vi "FancyPID.vi"(4 "Reset":bool, 6 "Gains":T1={"proportional gain (Kc)"=1.0, "integral time (Ti, min)"=0.01, "derivative time (Td, min)"=0.0} {"derivative time (Td, min)" format="%.3f"; "integral time (Ti, min)" format="%.3f"; "proportional gain (Kc)" format="%.3f"}, 7 "Range":cluster{"output high":dbl, "output low":dbl}={"output high"=0.6, "output low"=-0.6} {"output low" format="%.2f"; "output high" format="%.2f"}, 8 "Disable Range":dbl=0.5, 9 "Integral Range":dbl=25.0, 10 "Process variable":dbl, 11 "Setpoint":dbl) -> (3 "output":dbl format="%.2f")   [LabVIEW 2016]
uses:
  <vilib>/addons/control/pid/pid.llb/PID (DBL).vi
  <vilib>/addons/control/pid/NI_PID_pid.lvlib
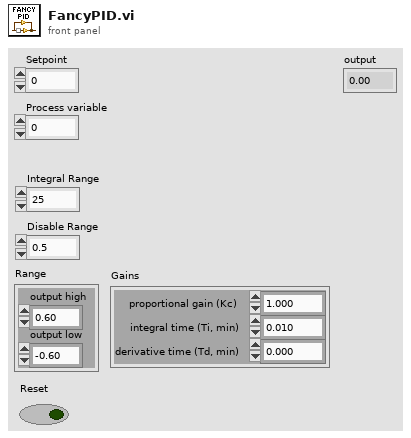
[diagram p1: front panel]
types:
  T1 = cluster{"proportional gain (Kc)":dbl, "integral time (Ti, min)":dbl, "derivative time (Td, min)":dbl}
  T2 = cluster{"proportional gain (Kc)":dbl, "f":dbl, "derivative time (Td, min)":dbl}
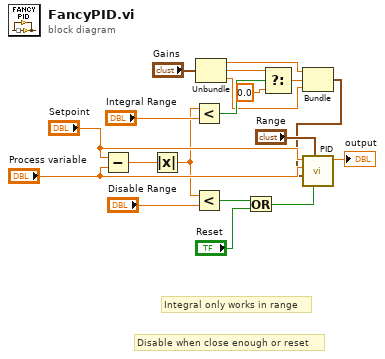
[diagram p0: block diagram]
diagram:
  # "Disable when close enough or reset"
  # "Integral only works in range"
  n1 = Subtract(x="Setpoint", y="Process variable") -> (x-y=w15:dbl)
  n2 = Absolute Value(x=w15) -> (abs(x)=w5:dbl)
  n3 = Less?(x=w5, y="Integral Range") -> (x < y?=w13:bool)
  n4 = Less?(x=w5, y="Disable Range") -> (x < y?=w3:bool)
  n5 = Unbundle("Gains") -> ("proportional gain (Kc)"=w8:dbl, "integral time (Ti, min)"=w11:dbl, "derivative time (Td, min)"=w7:dbl)
  n6 = Or(x=w3, y="Reset") -> (x .or. y?=w2:bool)
  n7 = Select(t=w11, s=w13, f=0.0) -> (s? t:f=w9:dbl)
  n8 = Bundle("proportional gain (Kc)"=w8, "f"=w9, "derivative time (Td, min)"=w7) -> (w1:T2)  [unwired: 1 in]
  n9 = call-poly <vilib>:"PID.vi"("reinitialize? (F)"=w2, "output range"="Range", "PID gains"=w1, "process variable"="Process variable", "setpoint"="Setpoint") -> ("output"=→"output":dbl)  [unwired: 5 in, 1 out]
